vi "ArrayFile.vi"(8 "error in":errorcluster caption="Error In", 10 "Array Size":i32, 11 "File Path":string) -> (0 "error out":errorcluster caption="Error Out", 3 "ArrayOut":dbl[](array[numeric]))   [LabVIEW 2014]
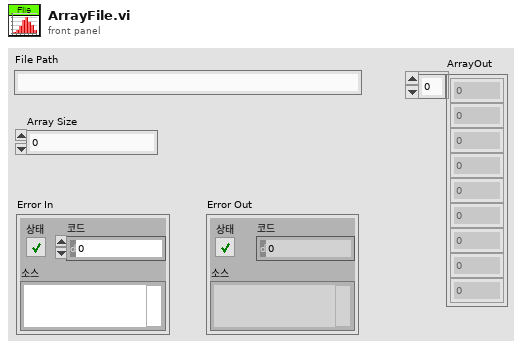
[diagram p1: front panel]
types:
  T1 = enum16{"open", "replace", "create", "open or create", "replace or create", "replace or create with confirmation"}
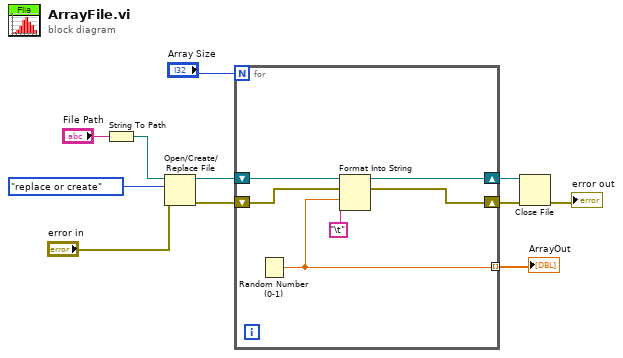
[diagram p0: block diagram]
diagram:
  n1 = String To Path(string="File Path") -> (path=w9:path)
  n2 = Open/Create/Replace File(file path (use dialog)=w9, error in="error in", operation (0:open)=T1."replace or create" ("동작(0:open)")) -> (refnum out=w6:refnum<file>, error out=w5:errorcluster)  [unwired: 3 in, 1 out]
  n3 = for {
    N: "Array Size" -> [_]
    shift-right: [w16] -> w3
    shift-left: w6 -> [w17]
    shift-right: [w14] -> w4
    shift-left: w5 -> [w15]
    tunnel: [w13] -> w1 mode=indexing
    n4 = Random Number (0-1)() -> (number: 0 to 1=w13:dbl)
    n5 = Format Into String(initial string=w17, error in=w15, w13, "\t") -> (resulting string=w16:refnum<file>, error out=w14:errorcluster)  [unwired: 1 in]
  }
  "ArrayOut" <- w1
  n6 = Close File(refnum=w3, error in=w4) -> (error out=→"error out":errorcluster)  [unwired: 1 out]
